vi "PID_SysLog.vi"(9 "Fehlermeldung":string, 10 "Boolesch":bool, 11 "Heizung\nFilterblock":T1 {"max. OUT" format="%#_5g"; "Regelzonengr." format="%#_5g"; "D-Anteil" format="%#_5g"; "I-Anteil" format="%#_5g"; "P-Anteil" format="%.1f"}) -> ()   [LabVIEW 2020, in "Erweiterte Konfig.lvlib"]
uses:
  Erweiterte Konfig.lvlib
  PID-Parameter.ctl
  Visualisierungs Elemente/Zahlen-Eingabefeld.ctl
  SysLog/SysLog Interface.ctl
  SysLog/SysLog.lvlib
panel:
  # "sec"
  # "sec"
  # "°C"
  # "%"
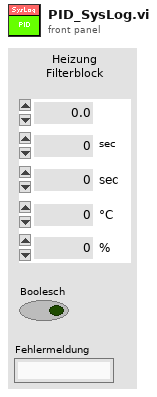
[diagram p1: front panel]
types:
  T1 = typedef "Erweiterte Konfig.lvlib/PID-Parameter.ctl" = cluster{"P-Anteil":T2, "I-Anteil":T2, "D-Anteil":T2, "Regelzonengr.":T2, "max. OUT":T2}
  T2 = typedef "Zahlen-Eingabefeld.ctl" = sgl
  T3 = typedef "SysLog.lvlib/SysLog Interface.ctl" = cluster{"Fehlermeldung":string, "Erfolgsmeldung":string, "Anzeige":bool, "SysLogIcon":enum16{"OK", "Warnung", "Fehler"}, "intern":bool}
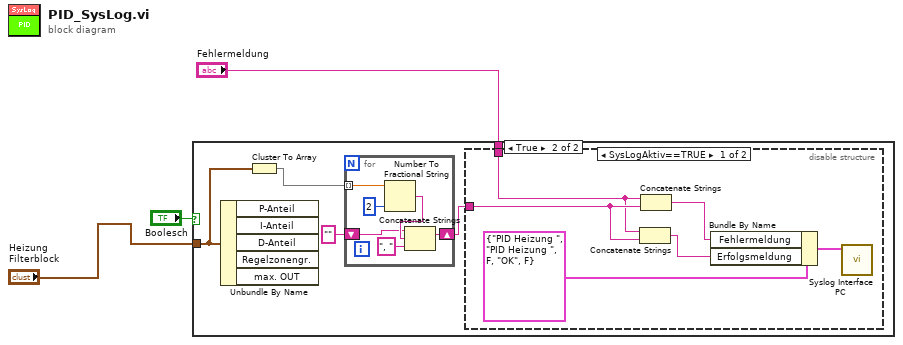
[diagram p0: block diagram]
diagram:
  n1 = case shown="True" "Boolesch" {
    tunnel: "Heizung\nFilterblock" -> [_ w8]
    tunnel: "Fehlermeldung" -> [_ w4]
    frame False {
    }
    frame True {
      n2 = Unbundle By Name(w8) -> ()  [unwired: 5 out]
      n3 = Cluster To Array(cluster=w8) -> (array=w7:T2[])
      n4 = for {
        tunnel: w7 -> [w14] mode=indexing
        shift-right: [w11] -> w5
        shift-left: "" -> [w12]
        n5 = Number To Fractional String(number=w14, precision (6)=i16 2 ("Genauigkeit (6)")) -> (F-format string=w13:string)  [unwired: 2 in]
        n6 = Concatenate Strings(w12, w13, ", " ("String")) -> (w11:string)
      }
      n7 = disable-structure shown="SysLogAktiv==TRUE" {
        disable-tunnel: w5 -> [w16 _]
        disable-tunnel: w4 -> [w15 _]
        frame condition #0 (active) {
          n8 = Concatenate Strings(w15, w16) -> (w17:string)
          n9 = Concatenate Strings(w15, w16) -> (w18:string)
          n10 = Bundle By Name(cluster=T3 {"Fehlermeldung"="PID Heizung ", "Erfolgsmeldung"="PID Heizung ", "Anzeige"=FALSE, "SysLogIcon"=enum."OK", "intern"=FALSE} ("Cluster (in)"), "Fehlermeldung"=w18, "Erfolgsmeldung"=w17) -> (w19:T3)
          n11 = call "Syslog Interface PC.vi"("Cluster (in)"=w19) -> ()  [unwired: 10 in, 1 out]
        }
        frame condition #1 {
        }
      }
    }
  }
